vi "Actor Core.vi"(8 "error in":errorcluster, 11 "Instr Actor in":refnum<class "Instr Actor.lvclass">) -> (0 "error out":errorcluster, 3 "Actor out":refnum<class "Actor.lvclass">)   [LabVIEW 2018, in "Instrument Library.lvlib" / "Instr Actor.lvclass"]
doc: "(<B>Filename</B>: Actor Framework.lvlib:Actor.lvclass:Actor Core.vi)\n\nReceives messages to the actor, reacts to them, and initiates any error handling that may shut the actor down.\n\nDescendant classes may override this VI to append parallel tasks for the actor to complete while it handles messages. Overrides use the Call Parent Method node."
uses:
  Instr Actor.lvclass
  <vilib>/ActorFramework/Actor/Actor.lvclass
  <vilib>/ActorFramework/Message Enqueuer/Message Enqueuer.lvclass
  reusable/DAQ Device/Device/Generic Data Update Data MSG/Generic Update Data Message.lvclass
  SuperActor/SuperActor.lvclass
  reusable/Instrument/Instrument.lvclass
  reusable/Session APIs/CVT/CVT.lvclass
  C:/Users/Labview/Documents/exscalabar_server/SuperActor/SuperActor.lvclass
  C:/Program Files (x86)/National Instruments/LabVIEW 2018/vi.lib/ActorFramework/Actor/Actor.lvclass
  C:/Program Files (x86)/National Instruments/LabVIEW 2018/vi.lib/ActorFramework/Message/Message.lvclass
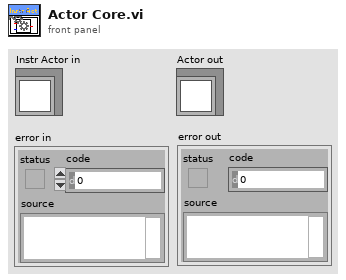
[diagram p1: front panel]
types:
  T1 = typedef "Session - Root.lvclass/Session Handle.ctl" = refnum<data-value>
  T2 = cluster{"tag":string, "section":string, "data":variant}
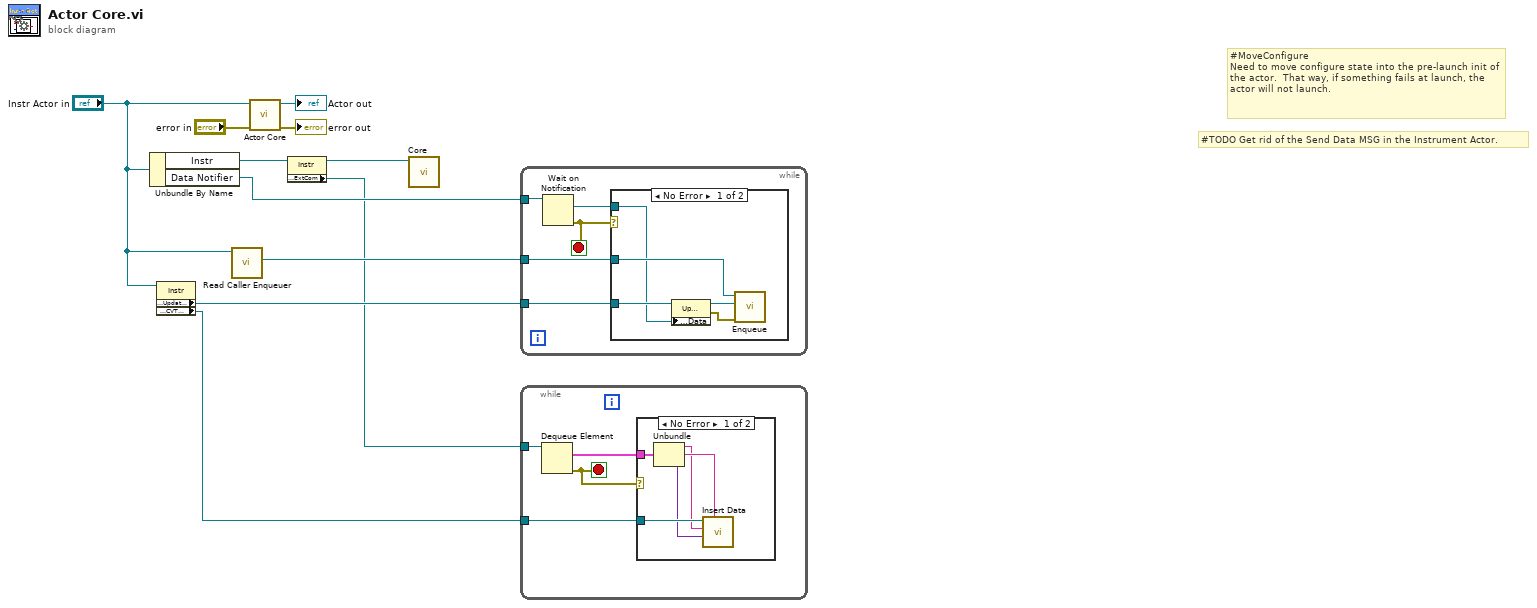
[diagram p0: block diagram]
diagram:
  # "#TODO Get rid of the Send Data MSG in the Instrument Actor."
  # "#MoveConfigure\nNeed to move configure state into the pre-launch init of the actor.  That way, if something fails at launch, the actor will not launch."
  n1 = Unbundle By Name("Instr Actor in") -> ("Instr"=w4:refnum<class "Instrument.lvclass">, "Data Notifier"=w8:refnum<notifier>)
  n2 = property class="Instr"(reference="Instr Actor in") -> ("Accessors:Update Data MSG"=w5:refnum<class "Generic Update Data Message.lvclass">, "Accessors:CVT Session"=w1:T1)  [unwired: 1 in, 2 out]
  n3 = call <vilib>:"Read Caller Enqueuer.vi"("Actor"="Instr Actor in") -> ("Caller Enqueuer"=w7:refnum<class "Message Enqueuer.lvclass">)  [unwired: 10 in]
  n4 = call-parent "Actor Core.vi"("error in"="error in", "Actor in"="Instr Actor in") -> ("error out"=→"error out":errorcluster, "Actor out"=→"Actor out":refnum<class "Actor.lvclass">)  [unwired: 8 in]
  n5 = property class="Instr"(reference=w4) -> (reference out=w3:refnum<class "Instrument.lvclass">, "Accessors:ExtCom"=w2:refnum<queue>)  [unwired: 1 in, 1 out]
  n6 = call "Core.vi"("Instr in"=w3) -> ()  [unwired: 11 in]
  n7 = while {
    tunnel: w8 -> [w16]
    tunnel: w7 -> [w15]
    tunnel: w5 -> [w12]
    stop <- w14 stop-if-true
    n8 = Wait on Notification(notifier=w16) -> (notification=w13:refnum<class "Data.lvclass">, error out=w14:errorcluster)  [unwired: 3 in, 2 out]
    n9 = case shown="No Error" w14 {
      tunnel: w15 -> [w21 _]
      tunnel: w13 -> [w18 _]
      tunnel: w12 -> [w20 _]
      frame No Error {
        n10 = property class="Update Data MSG"(reference=w20, "Accessors:Data"=w18) -> (reference out=w19:refnum<class "Generic Update Data Message.lvclass">, error out=w17:errorcluster)  [unwired: 1 in]
        n11 = call <vilib>:"Enqueue.vi"("error in (no error)"=w17, "Message"=w19, "Message Enqueuer in"=w21) -> ()  [unwired: 7 in, 2 out]
      }
      frame Error {
      }
    }
  }
  n12 = while {
    tunnel: w2 -> [w25]
    tunnel: w1 -> [w22]
    stop <- w24 stop-if-true
    n13 = Dequeue Element(queue=w25) -> (element=w23:T2, error out=w24:errorcluster)  [unwired: 2 in, 2 out]
    n14 = case shown="No Error" w24 {
      tunnel: w23 -> [w30 _]
      tunnel: w22 -> [w28 _]
      frame No Error {
        n15 = Unbundle(w30) -> ("tag"=w27:string, "section"=w29:string, "data"=w26:variant)
        n16 = call "Insert Data.vi"("Group"=w29, "Data"=w26, "tag"=w27, "CVT Session In"=w28) -> ()  [unwired: 6 in, 2 out]
      }
      frame Error {
      }
    }
  }
